vi "Read Stage Homed.vi"(8 "error in (no error)":errorcluster, 11 "2-Axis Stage Status in":refnum<class "2-Axis Stage Status.lvclass">) -> (0 "error out":errorcluster, 2 "Homed":bool, 3 "2-Axis Stage Status out":refnum<class "2-Axis Stage Status.lvclass">)   [LabVIEW 2022 SP3, in "2-Axis Stage Status.lvclass"]
uses:
  2-Axis Stage Status.lvclass
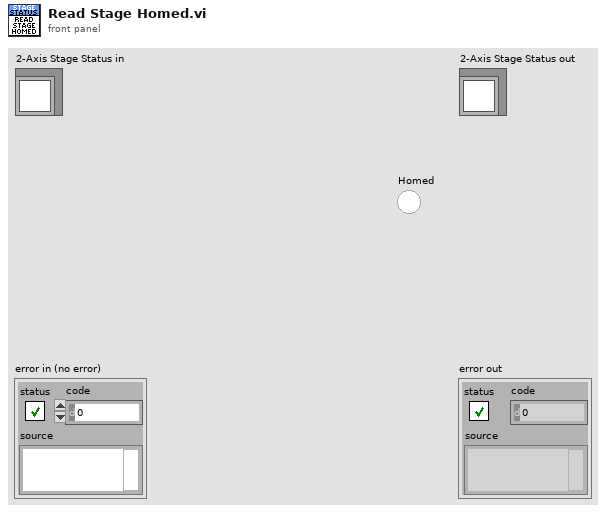
[diagram p1: front panel]
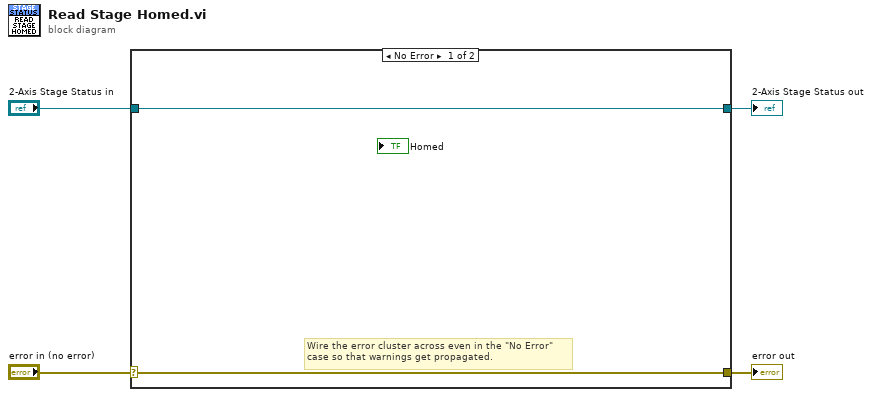
[diagram p0: block diagram]
diagram:
  n1 = case shown="No Error" "error in (no error)" {
    selector: "error in (no error)" -> [w5 w8]
    tunnel: [w5 w8] -> w3
    tunnel: [w6 w7] -> w1
    tunnel: "2-Axis Stage Status in" -> [w6 w7]
    frame No Error {
      # "Wire the error cluster across even in the \"No Error\"\ncase so that warnings get propagated."
    }
    frame Error {
    }
  }
  "error out" <- w3
  "2-Axis Stage Status out" <- w1
